vi "Read Quad Enc.vi"(0 "Clock":bool, 1 "Reset Enc":bool, 2 "A":bool, 3 "B":bool, 4 "Z":bool, 5 "Polarity":bool, 7 "Clock Divider":u16=1, 9 "Reset Position":i32) -> (14 "Vel/Acc Update":bool, 15 "Position (Counts)":i32, 16 "Velocity (Counts/Interval)":i32, 17 "Acceleration (Counts/Interval^2)":i32, 18 "dT (Ticks)":u32, 19 "CW Direction":bool)   [LabVIEW 2009]
doc: "Calculates 32-bit position, velocity, and acceleration based on a Quadrature encoder signal. This function resets the position upon the first Z index pulse. Subsequent Z index pulses are ignored. The velocity and acceleration values are not effected when the position is reset by the Z index pulse. The Direction input determines whether the function counts up or down based on clockwise motion.\n\nOPERATION\nUses A, B, and Z index signals to calculate position. Upon the falling edge of the Clock input, the function updates the position, velocity, acceleration, and elapsed time and latches the result. The velocity is calculated in units of Counts/Interval by subtracting the current position from the previous position. The acceleration is calculated in units of Counts/Interval^2 by subtracting the current velocity from the previous velocity.\n\nThe Clock Divider signal increases the time interval between velocity and acceleration estimates by N number of clocks to provide better resolution when the time interval between clock updates is small. Since more encoder counts are acquired during the time interval, the accuracy increases. The drawback is that the time delay also increases for the velocity and acceleration updates. The position always updates on every rising clock edge. If Clock Divider is set to 0 the Clock signal is ignored and the position, velocity, and acceleration are updated each time the function is called.\n\nThis function should be run as fast as possible to ensure that no Quadrature encoder digital edges are missed. Do not add delay timers into the loop containing this function.\n\nIf the encoder signals are noise, you may want to use the Filter Digital Lines, 3-ch (FPGA).vi function on the A, B, and Z signals before feeding them into this Quadrature encoder function.\n\nRT HOST INTERFACE\nIn your RT host application, you can divide Velocity (Counts/Interval) by the time interval dT (Ticks) to convert the velocity to units of Counts/Tick. By default, one tick is equal to 25 nanoseconds (40 MHz), so you can calculate the velocity in units of Counts per Second as follows,\n\nVelocity (Counts/s) = Velocity (Counts/Interval) / [dT (Ticks) * 25e-9 (s)]\n\nIn your RT host application, you can divide Acceleration (Counts/Interval^2) by the square of the time interval (dT (Ticks))^2 to convert the acceleration to units of Counts/Tick^2. By default, one tick is equal to 25 nanoseconds (40 MHz), so you can calculate the acceleration in units of Counts per Second^2 as follows,\n\nAcceleration (Counts/s^2) = Acceleration (Counts/Interval^2) / [(dT (Ticks))^2 * 25e-9^2 (s^2)]\n\nINPUTS\nClock- Falling edge latches the position, velocity, acceleration, and elapsed time\nReset- Sets the position to the Reset Position value\nA- Quadrature encoder A phase signal\nB- Quadrature encoder B phase signal\nZ- Quadrature encoder Z index signal\nPolarity- When FALSE, counterclockwise motion causes the Position (Counts) output to increment\nClock Divider- Causes the velocity and acceleration values to update every N clocks\nReset Position- The position will be set to this value when the first Z index pulse occurs or the Reset input is asserted\nVel/Acc Update- Boolean signal that changes state when the velocity and acceleration outputs are updated. Used for synchronization with other loops.\nCW Direction- If the Polarity input is FALSE, this signal is TRUE when clockwise motion is detected\n\n\nOUTPUTS\nPosition (Counts)- The position count value, updated continuously\nVelocity (Counts/Interval)- The amount the position has changed between the last two updates\nAcceleration (Counts/Interval^2)- The amount the velocity has changed between the last two updates\ndT (Ticks)- The time interval between velocity and acceleration updates, express in FPGA clock ticks\n\nNOTES\nBy allowing more time between updates you obtain more averaging on the velocity and acceleration values and therefore smoother results. A larger time interval results in less noise on the velocity and acceleration calculations. Also, using an encoder with more counts per revolution results in better accuracy and smoother results on the velocity and acceleration calculations.\n\nSaturation Subtract functions are used to saturate the signed velocity and acceleration values in the case of integer overflow. \n\nA normal Subtract function is used on the elapsed time counter. Because unsigned integers are used, the dT (Ticks) value is correct even when the Tick Count value rolls over."
uses:
  Instance           1 56Saved   Quadrature Encoder dX Method (FPGA, Use in SCTL) .vi
  Instance           2 56Saved   Quadrature Encoder dX Method (FPGA, Use in SCTL) .vi
  <vilib>/rvi/Arithmetic/AddSubMult/XNode/nirviSatArithmetic.xnode
panel:
  out "R9":u16
  out "R8":bool
  out "R7":u32
  out "R6":i32
  out "R5":i32
  out "R4":i32
  out "R3":bool
  out "R2":bool
  out "R1":bool
  # "Internal Registers"
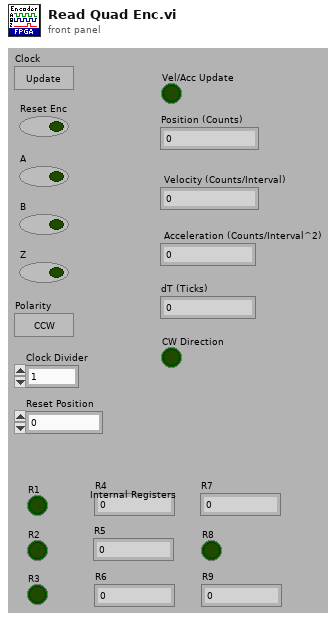
[diagram p1: front panel]
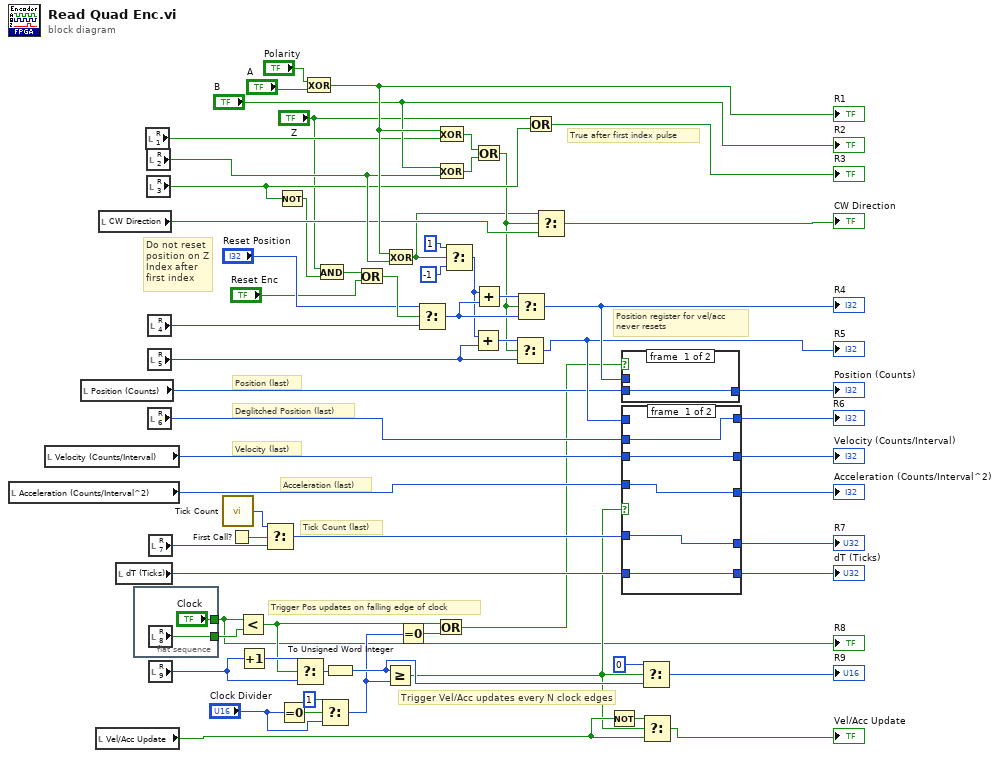
[diagram p0: block diagram]
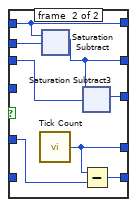
[diagram p3: hidden frame]
diagram:
  # "Trigger Vel/Acc updates every N clock edges"
  # "Trigger Pos updates on falling edge of clock"
  # "Position (last)"
  # "Tick Count (last)"
  # "Position register for vel/acc\nnever resets"
  # "True after first index pulse"
  # "Acceleration (last)"
  # "Velocity (last)"
  # "Deglitched Position (last)"
  # "Do not reset position on Z Index after first index"
  n1 = local read "Acceleration (Counts/Interval^2)"() -> (w41:i32)
  n2 = local read "Velocity (Counts/Interval)"() -> (w42:i32)
  n3 = local read "Position (Counts)"() -> (w44:i32)
  n4 = local read "Vel/Acc Update"() -> (w36:bool)
  n5 = local read "CW Direction"() -> (w47:bool)
  n6 = local read "dT (Ticks)"() -> (w39:u32)
  n7 = flat-sequence {
    tunnel: [w66] -> w38
    tunnel: ["Clock"] -> w1
    frame #0 {
      n8 = local read "R8"() -> (w66:bool)
    }
  }
  n9 = local read "R1"() -> (w50:bool)
  n10 = local read "R2"() -> (w49:bool)
  n11 = local read "R3"() -> (w48:bool)
  n12 = local read "R4"() -> (w46:i32)
  n13 = local read "R5"() -> (w45:i32)
  n14 = local read "R6"() -> (w43:i32)
  n15 = local read "R7"() -> (w40:u32)
  n16 = local read "R9"() -> (w37:u16)
  n17 = call "Tick Count"() -> ("Tick Count(Ticks)"=w6:u32)
  n18 = First Call?() -> (First Call?: T/F=w28:bool)
  n19 = Less?(x=w1, y=w38) -> (x < y?=w24:bool)
  n20 = Increment(x=w37) -> (x+1=w26:u16)
  n21 = Select(t=w6, s=w28, f=w40) -> (s? t:f=w27:u32)
  n22 = Not(x=w48) -> (.not. x?=w29:bool)
  n23 = Equal To 0?(x="Clock Divider") -> (x = 0?=w5:bool)
  n24 = Select(t=w26, s=w24, f=w37) -> (s? t:f=w25:u16)
  n25 = Exclusive Or(1:"A", 2:"Polarity") -> (0:w58:bool)
  "R1" <- w58
  n26 = And(x="Z", y=w29) -> (x .and. y?=w19:bool)
  n27 = Select(t=u16 1, s=w5, f="Clock Divider") -> (s? t:f=w2:u16)
  n28 = To Unsigned Word Integer(number=w25) -> (unsigned 16bit integer=w23:u16)
  n29 = Or(x=w19, y="Reset Enc") -> (x .or. y?=w18:bool)
  n30 = Greater Or Equal?(x=w23, y=w2) -> (x >= y?=w14:bool)
  n31 = Exclusive Or(1:w49, 2:w58) -> (0:w11:bool)
  n32 = Equal To 0?(x=w2) -> (x = 0?=w20:bool)
  n33 = Select(t="Reset Position", s=w18, f=w46) -> (s? t:f=w34:i32)
  n34 = Or(x=w24, y=w20) -> (x .or. y?=w21:bool)
  n35 = Exclusive Or(1:w50, 2:w58) -> (0:w30:bool)
  n36 = Exclusive Or(1:w49, 2:"B") -> (0:w31:bool)
  n37 = Select(t=1 ("32 bit"), s=w11, f=-1 ("32 bit")) -> (s? t:f=w16:i32)
  n38 = Add(x=w16, y=w45) -> (x+y=w17:i32)
  n39 = Or(x=w30, y=w31) -> (x .or. y?=w12:bool)
  n40 = Add(x=w16, y=w34) -> (x+y=w35:i32)
  n41 = Select(t=w17, s=w12, f=w45) -> (s? t:f=w54:i32)
  "R5" <- w54
  n42 = Select(t=w35, s=w12, f=w34) -> (s? t:f=w55:i32)
  "R4" <- w55
  n43 = Or(x="Z", y=w48) -> (x .or. y?=→"R3":bool)
  n44 = Select(t=w11, s=w12, f=w47) -> (s? t:f=→"CW Direction":bool)
  n45 = Not(x=w36) -> (.not. x?=w15:bool)
  n46 = case shown="False" w21 {
    tunnel: w55 -> [_ w68]
    tunnel: w44 -> [w67 _]
    tunnel: [w67 w68] -> w64
    frame #0 {
    }
    frame #1 {
    }
  }
  "Position (Counts)" <- w64
  n47 = case shown="True" w14 {
    tunnel: w54 -> [_ w81]
    tunnel: [w73 w81] -> w53
    tunnel: w43 -> [w73 w80]
    tunnel: [w72 w79] -> w63
    tunnel: w42 -> [w72 w78]
    tunnel: [w71 w77] -> w62
    tunnel: w41 -> [w71 _]
    tunnel: [w70 w76] -> w61
    tunnel: w39 -> [w70 _]
    tunnel: [w69 w75] -> w52
    tunnel: w27 -> [w69 w74]
    frame #0 {
    }
    frame #1 {
      n48 = call "Tick Count"() -> ("Tick Count(Ticks)"=w75:u32)
      n49 = xnode ("Saturation Subtract")("x"=w81, "y"=w80) -> ("x-y"=w79:i32)
      n50 = Subtract(x=w75, y=w74) -> (x-y=w76:u32)
      n51 = xnode ("Saturation Subtract3")("x"=w79, "y"=w78) -> ("x-y"=w77:i32)
    }
  }
  "Velocity (Counts/Interval)" <- w63
  "Acceleration (Counts/Interval^2)" <- w62
  "dT (Ticks)" <- w61
  "R6" <- w53
  "R7" <- w52
  n52 = Select(t=u16 0, s=w14, f=w23) -> (s? t:f=→"R9":u16)
  n53 = Select(t=w15, s=w14, f=w36) -> (s? t:f=→"Vel/Acc Update":bool)
  "R2" <- "B"
  "R8" <- w1
